vi "Simulation Time Elapsed.vi"(8 "error in (no error)":errorcluster, 11 "Time Target (s)":sgl) -> (0 "error out":errorcluster, 2 "dt (s)":dbl, 3 "Time Elapsed?":bool)   [LabVIEW 2013]
uses:
  <vilib>/robotics/Simulator/Interface/Simulator References/Get World Reference.vi
  <vilib>/robotics/Simulator/NI_Robotics_Simulator.lvlib
  <resource>/objmgr/LVODE.rc
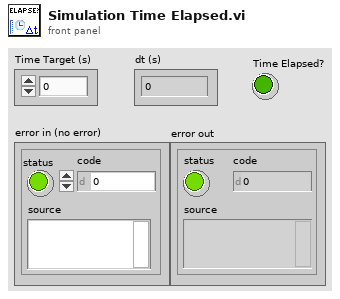
[diagram p1: front panel]
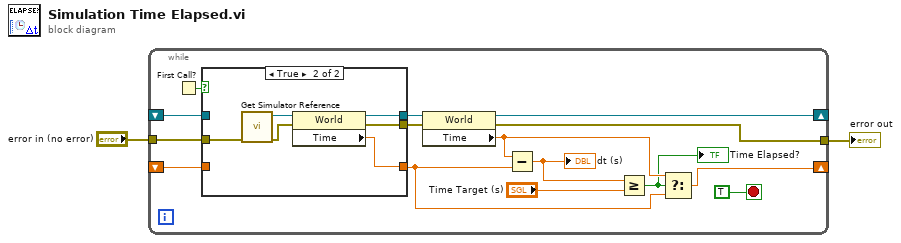
[diagram p0: block diagram]
diagram:
  n1 = while {
    tunnel: "error in (no error)" -> [w16]
    tunnel: [w10] -> w1
    shift-right: [w11] -> _
    shift-left: _ -> [w15]
    shift-right: [w5] -> _
    shift-left: _ -> [w14]
    stop <- TRUE stop-if-true
    n2 = First Call?() -> (First Call?: T/F=w17:bool)
    n3 = case shown="True" w17 {
      tunnel: [w18 w24] -> w12
      tunnel: w16 -> [w18 w23]
      tunnel: [w20 w22] -> w13
      tunnel: w15 -> [w20 _]
      tunnel: [w19 w21] -> w6
      tunnel: w14 -> [w19 _]
      frame False {
      }
      frame True {
        n4 = call-poly <vilib>:"Get Simulator Reference.vi"("error in (no error)"=w23) -> ("error out"=w25:errorcluster, "world ref"=w26:refnum<k20>)  [unwired: 9 in]
        n5 = property class="World"(reference=w26, error in=w25) -> (reference out=w22:refnum<k20>, error out=w24:errorcluster, "Time"=w21:sgl)
      }
    }
    n6 = property class="World"(reference=w13, error in=w12) -> (reference out=w11:refnum<k20>, error out=w10:errorcluster, "Time"=w7:sgl)
    n7 = Subtract(x=w7, y=w6) -> (x-y=w3:sgl)
    "dt (s)" <- w3
    n8 = Greater Or Equal?(x=w3, y="Time Target (s)") -> (x >= y?=w4:bool)
    "Time Elapsed?" <- w4
    n9 = Select(t=w7, s=w4, f=w6) -> (s? t:f=w5:sgl)
  }
  "error out" <- w1
